vi "cycle.vi"(0 "iteration":i32) -> (4 "message":string)   [LabVIEW 2026]
doc: "A plug for the Timed Loop slot template. Same connector pane as alternate.vi - iteration in, message out - but it reports the cycle number instead of alternating a fixed text, which is what makes it proof that the slot takes arbitrary content."
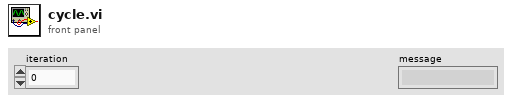
[diagram p1: front panel]
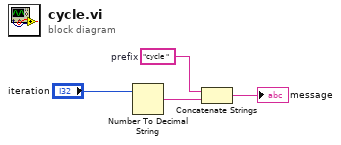
[diagram p0: block diagram]
diagram:
  w3 = "cycle "  # prefix
  n1 = Number To Decimal String(number="iteration") -> (decimal integer string=w2:string)  [unwired: 1 in]
  n2 = Concatenate Strings(w3, w2) -> (→"message":string)
